vi "Time Stamp.vi"(1 "Action":T2=enum."Identify", 2 "Parameters":variant) -> (6 "Output":variant, 7 "Stop":bool)   [LabVIEW 2021]
uses:
  Sub Controls/Instrument Actions.ctl
  Sub Controls/Public.ctl
  Sub Controls/Scan Output.ctl
  Sub Controls/User Event Command.ctl
panel:
  in  "Relative":enum32{"Relative Time", "Absolute Time"}(radio)
  out "Title":string="Timestamp"
  in  "Output?":bool=TRUE
  in  "Delay Time (Seconds)":dbl min=0.0 max=1000.0 format="%.1g"
  in  "Public":T1
  out "Measurement":dbl format="%.2g"
  in  "Index":i32
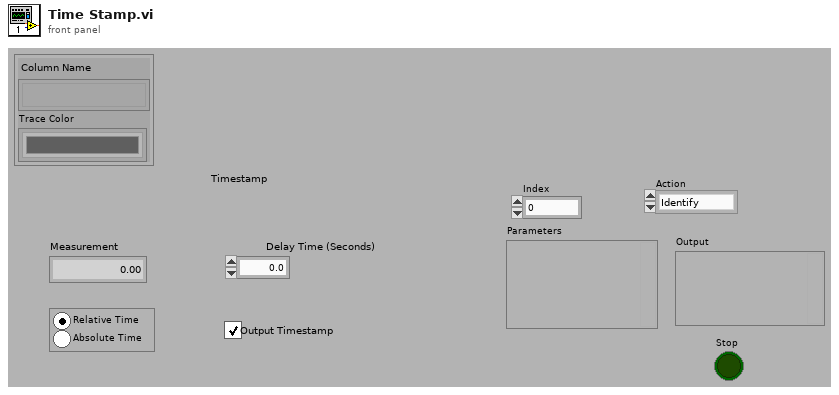
[diagram p1: front panel]
types:
  T1 = typedef "Public.ctl" = cluster{"Column Name":string[], "Trace Color":u32[]}
  T2 = typedef "Instrument Actions.ctl" = enum16{"Scan", "Identify", "New", "Configure", "Initialize", "Test", "Read", "Close"}
  T3 = typedef "Scan Output.ctl" = cluster{"Manufacturer":string, "Model":string, "Info":string, "Revision":string, "error out":errorcluster}
  T4 = typedef "User Event Command.ctl" = enum32{"Stop Config"}
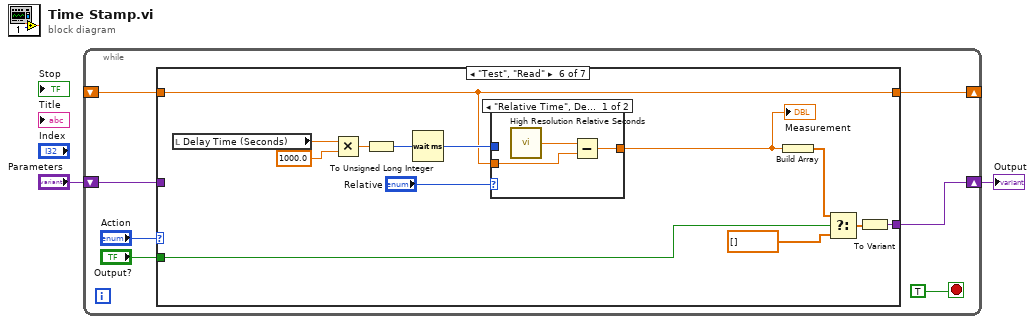
[diagram p0: block diagram]
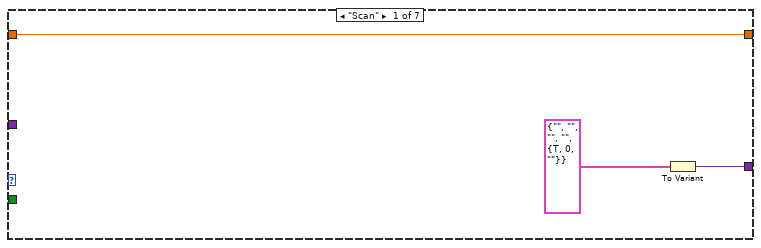
[diagram p2: hidden frame]
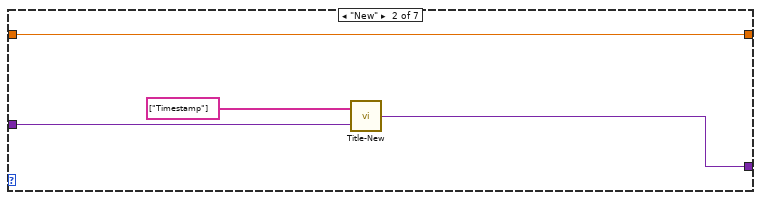
[diagram p3: hidden frame]
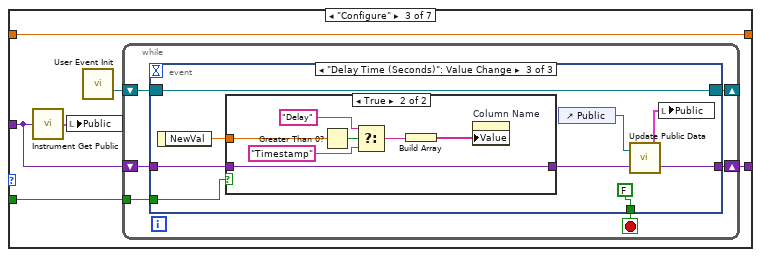
[diagram p4: hidden frame]
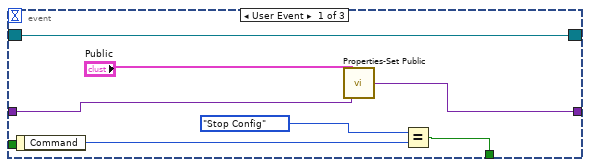
[diagram p5: hidden frame]
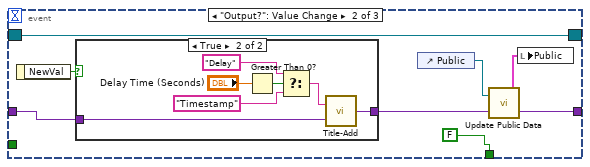
[diagram p6: hidden frame]
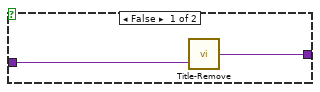
[diagram p7: hidden frame]
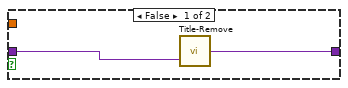
[diagram p8: hidden frame]
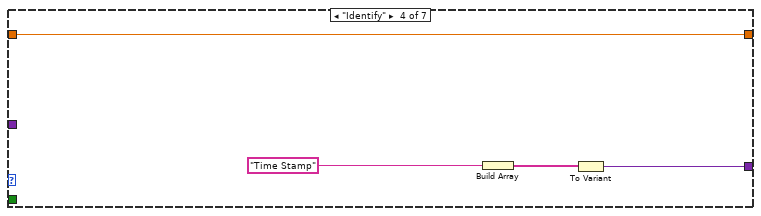
[diagram p9: hidden frame]
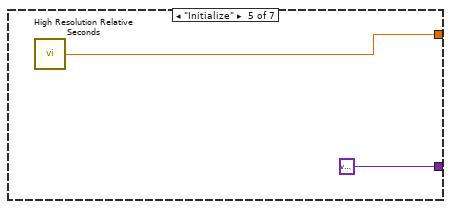
[diagram p10: hidden frame]
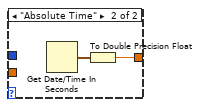
[diagram p11: hidden frame]
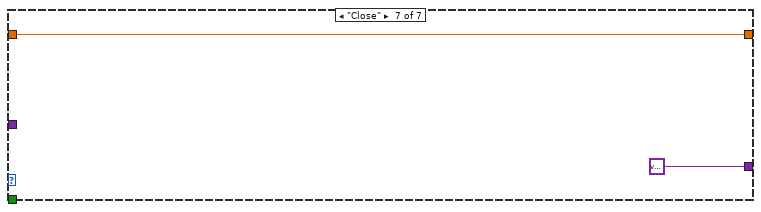
[diagram p12: hidden frame]
diagram:
  n1 = while {
    shift-right: [w8] -> _
    shift-left: _ -> [w7]
    shift-right: [w5] -> w1
    shift-left: "Parameters" -> [w6]
    stop <- TRUE stop-if-true
    n2 = case shown="\"Test\", \"Read\"" "Action" {
      tunnel: [w11 w15 w22 w72 w76 w79 w96] -> w8
      tunnel: w7 -> [w11 w15 w22 w72 _ w79 w96]
      tunnel: w6 -> [_ w16 w19 _ _ _ _]
      tunnel: [w10 w13 w21 w71 variant ("Variant") w89 variant ("Variant")] -> w5
      tunnel: "Output?" -> [_ _ w17 _ _ w81 _]
      frame "Scan" {
        n3 = To Variant(anything=T3 {"Manufacturer"="", "Model"="", "Info"="", "Revision"="", "error out"={"status"=TRUE, "code"=0, "source"=""}} ("Scan Output")) -> (Variant=w10:variant)
      }
      frame "New" {
        n4 = call "Title-New.vi"("Parameters"=w16, "Array"=string[] ["Timestamp"]) -> ("Instrument Prop"=w13:variant)
      }
      frame "Configure" {
        n5 = call "Instrument Get Public.vi"("Variant"=w19) -> ("Public"=w20:T1)
        n6 = local write "Public"(w20) -> ()
        n7 = call "User Event Init.vi"() -> ("Event Registration Refnum"=w18:refnum<event-registration>)  [unwired: 14 in, 1 out]
        n8 = while {
          shift-right: [w28] -> w21
          shift-left: w19 -> [w27]
          shift-right: [w24] -> _
          shift-left: w18 -> [w25]
          tunnel: w17 -> [w23]
          stop <- w26 stop-if-true
          n9 = event shown="[2] \"Delay Time (Seconds)\": Value Change" {
            selector: w25 -> [w29 w41 w60]
            dyn-events: [w29 w41 w60] -> w24
            timeout: _ -> [_ _ _]
            tunnel: [w31 FALSE FALSE] -> w26
            tunnel: w27 -> [w34 w42 w61]
            tunnel: [w35 w39 w58] -> w28
            tunnel: w23 -> [_ _ w53]
            event User Event {
              n10 = event-data() -> ("Command"=w33:T4)  [unwired: 1 in]
              n11 = call "Properties-Set Public.vi"("Variant"=w34, "New Public"="Public") -> ("Variant 2"=w35:variant)
              n12 = Equal?(x=User_Event_Command."Stop Config", y=w33) -> (x = y?=w31:bool)
            }
            event "Output?": Value Change {
              n13 = event-data() -> ("NewVal"=w43:bool)  [unwired: 1 in]
              n14 = case shown="True" w43 {
                tunnel: w42 -> [w45 w52]
                tunnel: [w44 w51] -> w40
                frame False {
                  n15 = call "Title-Remove.vi"("Parameters"=w45) -> ("Variant"=w44:variant)  [unwired: 1 in]
                }
                frame True {
                  n16 = Greater Than 0?(x="Delay Time (Seconds)") -> (x > 0?=w48:bool)
                  n17 = Select(t="Delay" ("String"), s=w48, f="Timestamp" ("String")) -> (s? t:f=w47:string)
                  n18 = call "Title-Add.vi"("Parameters"=w52, "String"=w47) -> ("Variant"=w51:variant)
                }
              }
              n19 = control-ref of="Public"() -> (w37:refnum<vi>)
              n20 = call "Update Public Data.vi"("Variant In"=w40, "Public 2"=w37) -> ("Variant Out"=w39:variant, "Public"=w38:T1)
              n21 = local write "Public"(w38) -> ()
            }
            event "Delay Time (Seconds)": Value Change {
              n22 = event-data() -> ("NewVal"=w54:dbl)  [unwired: 1 in]
              n23 = case shown="True" w53 {
                tunnel: w61 -> [w63 w66]
                tunnel: [w62 w66] -> w59
                tunnel: w54 -> [_ w67]
                frame False {
                  n24 = call "Title-Remove.vi"("Parameters"=w63) -> ("Variant"=w62:variant)  [unwired: 1 in]
                }
                frame True {
                  n25 = Greater Than 0?(x=w67) -> (x > 0?=w68:bool)
                  n26 = Select(t="Delay" ("String"), s=w68, f="Timestamp" ("String")) -> (s? t:f=w65:string)
                  n27 = Build Array(w65) -> (w64:string[])
                  n28 = property on="Column Name" class="Arr (strict)"("Value"=w64) -> ()  [unwired: 2 in, 2 out]
                }
              }
              n29 = control-ref of="Public"() -> (w56:refnum<vi>)
              n30 = call "Update Public Data.vi"("Variant In"=w59, "Public 2"=w56) -> ("Variant Out"=w58:variant, "Public"=w57:T1)
              n31 = local write "Public"(w57) -> ()
            }
          }
        }
      }
      frame "Identify" {
        n32 = Build Array("Time Stamp") -> (w74:string[])
        n33 = To Variant(anything=w74) -> (Variant=w71:variant)
      }
      frame "Initialize" {
        n34 = call <vilib>:"High Resolution Relative Seconds.vi"() -> ("relative seconds"=w76:dbl)
      }
      frame "Test", "Read" {
        n35 = local read "Delay Time (Seconds)"() -> (w87:dbl)
        n36 = Multiply(x=w87, y=1000.0 ("x")) -> (x*y=w88:dbl)
        n37 = To Unsigned Long Integer(number=w88) -> (unsigned 32bit integer=w86:u32)
        n38 = Wait (ms)(milliseconds to wait=w86) -> (millisecond timer value=w80:u32)
        n39 = case shown="\"Relative Time\", Default" "Relative" {
          tunnel: w80 -> [_ _]
          tunnel: w79 -> [w92 _]
          tunnel: [w90 w93] -> w78
          frame "Relative Time", Default {
            n40 = call <vilib>:"High Resolution Relative Seconds.vi"() -> ("relative seconds"=w91:dbl)
            n41 = Subtract(x=w91, y=w92) -> (x-y=w90:dbl)
          }
          frame "Absolute Time" {
            n42 = Get Date/Time In Seconds() -> (seconds since 1Jan1904=w94:timestamp)
            n43 = To Double Precision Float(number=w94) -> (double precision float=w93:dbl)
          }
        }
        "Measurement" <- w78
        n44 = Build Array(w78) -> (w83:dbl[])
        n45 = Select(t=w83, s=w81, f=dbl[] []) -> (s? t:f=w84:dbl[])
        n46 = To Variant(anything=w84) -> (Variant=w89:variant)
      }
      frame "Close" {
      }
    }
  }
  "Output" <- w1
